vi "load cache into FGV.vi"(11 "classes":T1[](array[typedef])) -> ()   [LabVIEW 2013, in "PL_class cache.lvlib"]
uses:
  PL_class cache.lvlib
  class metadata.ctl
  class type.ctl
  class FGV actions.ctl
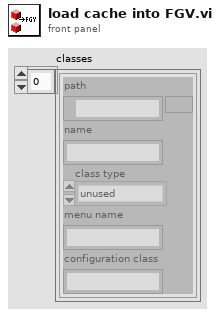
[diagram p1: front panel]
types:
  T1 = typedef "PL_class cache.lvlib/class metadata.ctl" = cluster{"path":path, "name":string, "class type":T2, "menu name":string, "configuration class":string}
  T2 = typedef "PL_class cache.lvlib/class type.ctl" = enum16{"unused", "other pl", "system", "target", "engine", "module"}
  T3 = typedef "PL_class cache.lvlib/class FGV actions.ctl" = enum16{"Add Element to Type", "Write Type", "Read  Type", "Read All", "Init"}
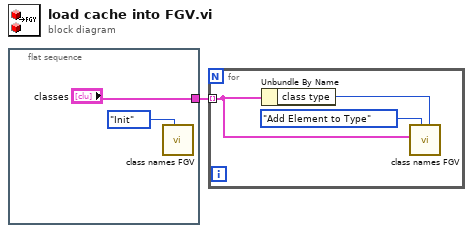
[diagram p0: block diagram]
diagram:
  n1 = flat-sequence {
    tunnel: ["classes"] -> w1
    frame #0 {
      n2 = call "class names FGV.vi"("Action"=class_FGV_actions."Init") -> ()  [unwired: 10 in, 1 out]
    }
  }
  n3 = for {
    tunnel: w1 -> [w4] mode=indexing
    n4 = Unbundle By Name(w4) -> ("class type"=w5:T2)
    n5 = call "class names FGV.vi"("class type"=w5, "Action"=class_FGV_actions."Add Element to Type", "class metadata"=w4) -> ()  [unwired: 8 in, 1 out]
  }
